vi "Format Live Data.vi"(10 "Live DI Data":u32[](array[numeric])=[0, 0, 0]) -> (2 "Array":i16[](array[numeric]))   [LabVIEW 2017]
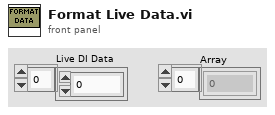
[diagram p1: front panel]
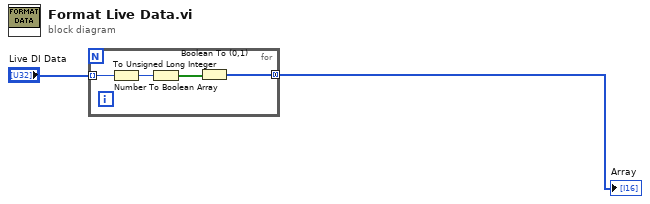
[diagram p0: block diagram]
diagram:
  n1 = for {
    tunnel: "Live DI Data" -> [w5] mode=indexing
    tunnel: [w3] -> w2 mode=concatenating
    n2 = To Unsigned Long Integer(number=w5) -> (unsigned 32bit integer=w4:u32)
    n3 = Number To Boolean Array(number=w4) -> (Boolean array=w6:bool[])
    n4 = Boolean To (0,1)(Boolean=w6) -> (0, 1=w3:i16[])
  }
  "Array" <- w2
